vi "Read-write Ini file.vi"(9 "OPERATION":u16(ring) items=["Write", "Read"], 10 "LAST DATA FILE":path) -> (2 "LAST DATA FILE 2":path)   [LabVIEW 2018]
panel:
  out "string":string
  out "path":path
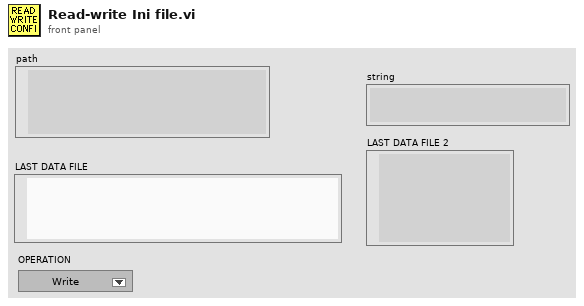
[diagram p1: front panel]
types:
  T1 = enum16{"open", "replace", "create", "open or create", "replace or create", "replace or create with confirmation"}
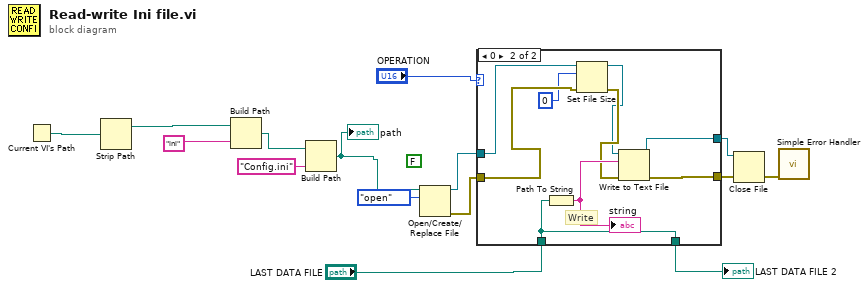
[diagram p0: block diagram]
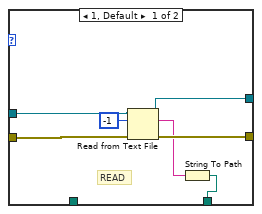
[diagram p2: hidden frame]
diagram:
  (unwired) FALSE ("create file if necessary (T)")
  n1 = Current VI's Path() -> (path=w15:path)
  n2 = Strip Path(path=w15) -> (stripped path=w14:path)  [unwired: 1 out]
  n3 = Build Path(base path=w14, name or relative path="ini" ("element")) -> (appended path=w12:path)
  n4 = Build Path(base path=w12, name or relative path="Config.ini" ("element")) -> (appended path=w6:path)
  "path" <- w6
  n5 = Open/Create/Replace File(file path (use dialog)=w6, operation (0:open)=T1."open") -> (refnum out=w4:refnum<file>, error out=w5:errorcluster)  [unwired: 4 in, 1 out]
  n6 = case shown="0" "OPERATION" {
    tunnel: w4 -> [w19 w26]
    tunnel: w5 -> [w22 w27]
    tunnel: [w21 w31] -> w10
    tunnel: [w20 w30] -> w2
    tunnel: "LAST DATA FILE" -> [_ w28]
    tunnel: [w18 w28] -> w1
    frame 1, Default {
      # "READ"
      n7 = Read from Text File(file (use dialog)=w19, count=-1, error in=w22) -> (refnum out=w20:refnum<file>, text=w17:string, error out=w21:errorcluster)  [unwired: 1 in, 1 out]
      n8 = String To Path(string=w17) -> (path=w18:path)
    }
    frame 0 {
      # "Write"
      n9 = Path To String(path=w28) -> (string=w29:string)
      "string" <- w29
      n10 = Set File Size(4:w27, 6:i64 0 ("offset (in bytes) (0)"), 7:w26) -> (0:w24:errorcluster, 3:w23:refnum<file>)
      n11 = Write to Text File(file (use dialog)=w23, text=w29, error in=w24) -> (refnum out=w30:refnum<file>, error out=w31:errorcluster)  [unwired: 1 in, 1 out]
    }
  }
  "LAST DATA FILE 2" <- w1
  n12 = Close File(refnum=w2, error in=w10) -> (error out=w7:errorcluster)  [unwired: 1 out]
  n13 = call <vilib>:"Simple Error Handler.vi"("error in (no error)"=w7) -> ()  [unwired: 4 in, 5 out]
